vi "HEWH Populate Test Pattern Cluster.vi"(8 "Error In":errorcluster, 11 "all rows":string[][](array[string])) -> (0 "Error Out":errorcluster, 3 "Cluster":T1={"Sequence #"=0.0, "Cycles"=0, "Mode Setting"="", "Flow Rate (GPM)"=0.0, "Temperature (F)"=0.0, "Reset Timer"=FALSE, "Use Temp Decline Method"=FALSE, "Terminate Condition"=enum."C1-Terminate Draw @ Gallon Mark", "Condition Value #1"=0.0, "UE"=FALSE, "LE"=FALSE, "Comp"=FALSE, "Fan"=FALSE, "Test End Time (Sec)"=0.0, "Purge Until Cutout"=FALSE, "Start Conditions"=enum."Heat Source Cutout", "Condition Value #2"=0.0, "Remove Power"=FALSE, "Time"=0.0, "Check Special Cond."=enum."SC1-Do Nothing", "Condition#"=enum."C1", "Draw Flags"=enum."N/A", "Data Processing Delay (FHD 15sec, UEF 5 Sec)"=0.0, "Test Complete"=FALSE} {"Time" format="%<%H:%M:%S>t"})   [LabVIEW 2016]
uses:
  Type Definitions/PRAT Test.ctl
  Utility/Save File/File Setup (Public)/Type Definition/Save File HEWH Heating Control Mode.ctl
  Draw Water Specific/Type Definitions/Terminate Draw Conditions.ctl
  Type Definitions/HEWH Start Conditions.ctl
  Draw Water Specific/Type Definitions/Check Special Condtions.ctl
  Draw Water Specific/Type Definitions/HEWH Special Condition Check.ctl
  Type Definitions/HEWH Draw Flag ENUM.ctl
  Utility/Save File/File Setup.lvlib
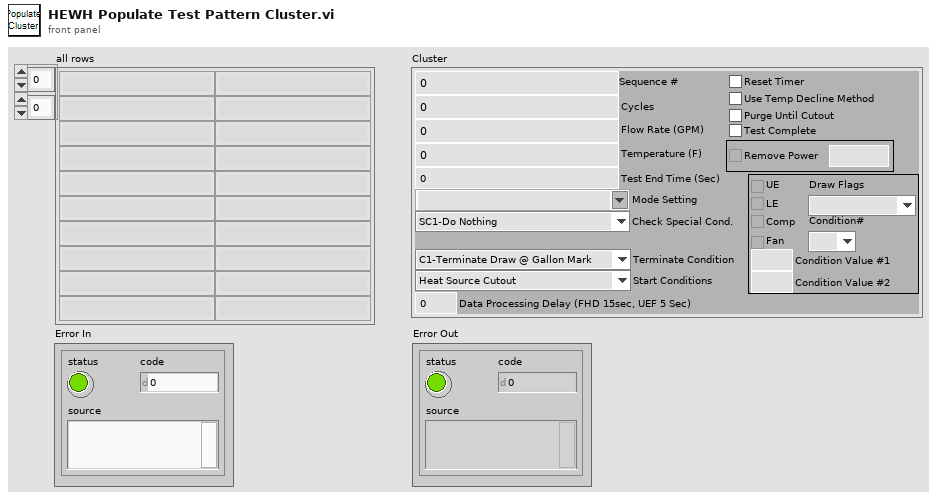
[diagram p1: front panel]
types:
  T1 = typedef "PRAT Test.ctl" = cluster{"Sequence #":dbl, "Cycles":i32, "Mode Setting":T2, "Flow Rate (GPM)":dbl, "Temperature (F)":dbl, "Reset Timer":bool, "Use Temp Decline Method":bool, "Terminate Condition":T3, "Condition Value #1":dbl, "UE":bool, "LE":bool, "Comp":bool, "Fan":bool, "Test End Time (Sec)":dbl, "Purge Until Cutout":bool, "Start Conditions":T4, "Condition Value #2":dbl, "Remove Power":bool, "Time":dbl, "Check Special Cond.":T5, "Condition#":T6, "Draw Flags":T7, "Data Processing Delay (FHD 15sec, UEF 5 Sec)":dbl, "Test Complete":bool}
  T2 = typedef "File Setup.lvlib/Save File HEWH Heating Control Mode.ctl" = string
  T3 = typedef "Terminate Draw Conditions.ctl" = enum16{"C1-Terminate Draw @ Gallon Mark", "C2-Special Last Draw (HU Test)", "C3-RTD Out <=", "C4-Mean Tank Temp <=", "C5-Decrease RTD Out (Deg F)", "C6-Time (Seconds)", "C7-Until Any Heat Source", "C8-Specific Heat Source", "C9-Do Nothing"}
  T4 = typedef "HEWH Start Conditions.ctl" = enum16{"Heat Source Cutout", "At Time (Seconds)", "Every X (Seconds)", "T2 >= X° Below Setpoint", "Seconds From Complete", "Wait for LE & Comp Cutout", "Wait for Comp Cutout", "Wait for LE Cutout", "Wait for UE Cutout"}
  T5 = typedef "Check Special Condtions.ctl" = enum16{"SC1-Do Nothing", "SC2-Check Heat Source (On-C2/Off-C1)", "SC3-Check Skip Condition", "SC4-Check Heat Source ON/Fail"}
  T6 = typedef "HEWH Special Condition Check.ctl" = enum16{"N/A", "C1", "C2", "Reset/Fail", "Skip Draw Sequence"}
  T7 = typedef "HEWH Draw Flag ENUM.ctl" = enum16{"N/A", "None(0)", "Sml(1)", "Med(2)", "SmlMed(3)", "Lrg(4)", "SmlLrg(5)", "MedLrg(6)", "SmlMedLrg(7)"}
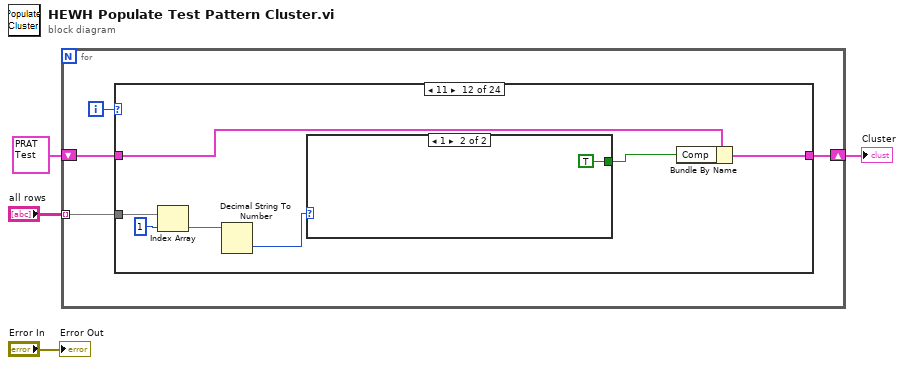
[diagram p0: block diagram]
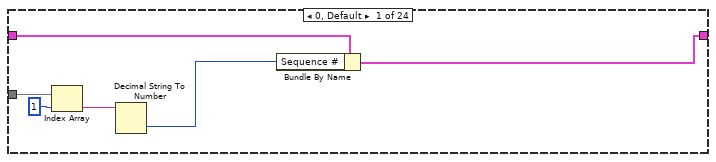
[diagram p2: hidden frame]
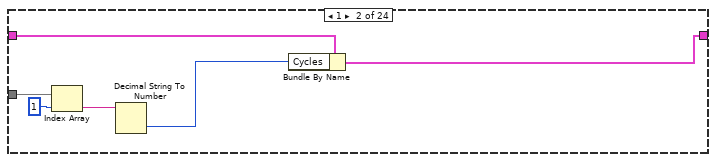
[diagram p3: hidden frame]
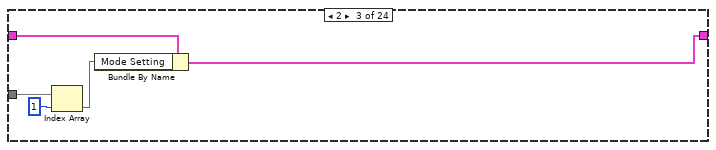
[diagram p4: hidden frame]
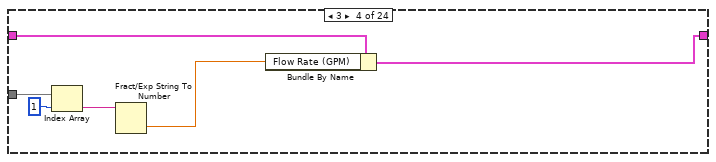
[diagram p5: hidden frame]
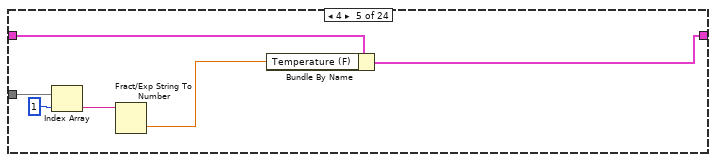
[diagram p6: hidden frame]
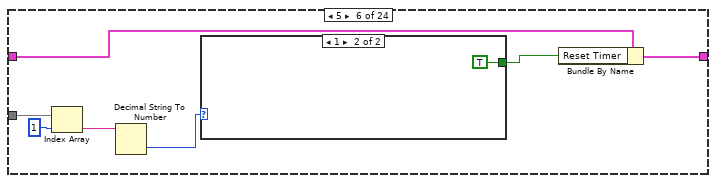
[diagram p7: hidden frame]
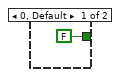
[diagram p8: hidden frame]
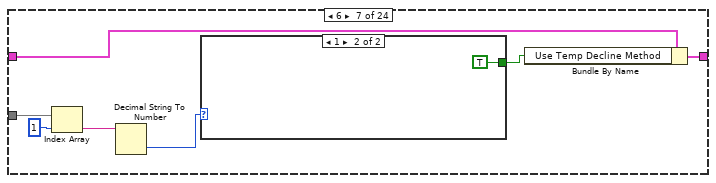
[diagram p9: hidden frame]
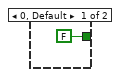
[diagram p10: hidden frame]
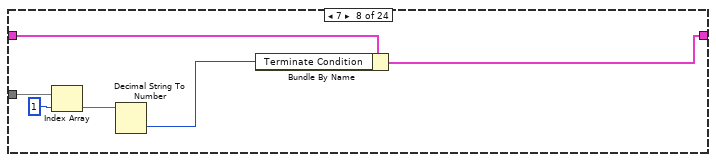
[diagram p11: hidden frame]
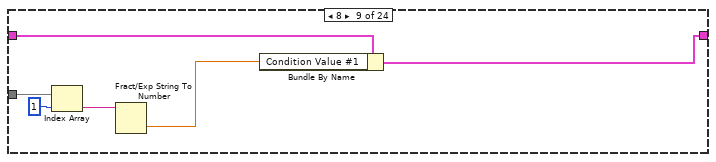
[diagram p12: hidden frame]
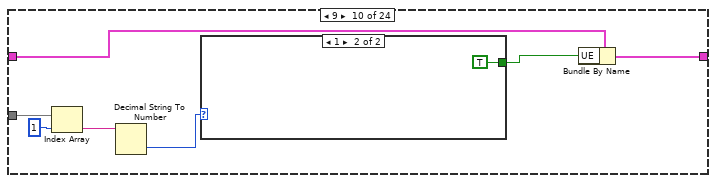
[diagram p13: hidden frame]
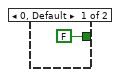
[diagram p14: hidden frame]
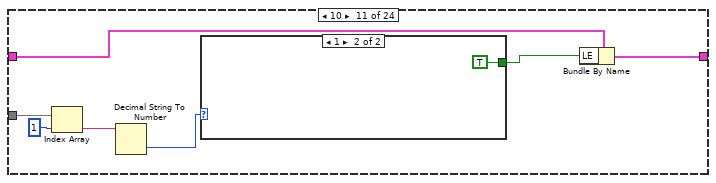
[diagram p15: hidden frame]
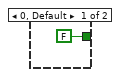
[diagram p16: hidden frame]
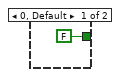
[diagram p17: hidden frame]
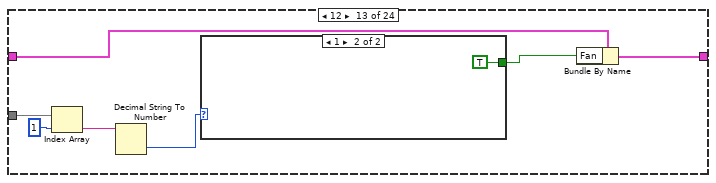
[diagram p18: hidden frame]
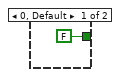
[diagram p19: hidden frame]
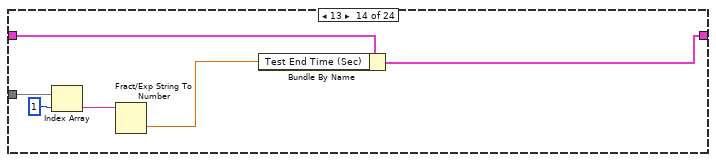
[diagram p20: hidden frame]
diagram:
  n1 = for {
    tunnel: "all rows" -> [w5] mode=indexing
    shift-right: [w6] -> w3
    shift-left: T1 {"Sequence #"=1.0, "Cycles"=1, "Mode Setting"="", "Flow Rate (GPM)"=3.0, "Temperature (F)"=58.0, "Reset Timer"=FALSE, "Use Temp Decline Method"=FALSE, "Terminate Condition"=enum."C9-Do Nothing", "Condition Value #1"=0.0, "UE"=FALSE, "LE"=FALSE, "Comp"=FALSE, "Fan"=FALSE, "Test End Time (Sec)"=0.0, "Purge Until Cutout"=FALSE, "Start Conditions"=enum."Heat Source Cutout", "Condition Value #2"=0.0, "Remove Power"=FALSE, "Time"=82800.0, "Check Special Cond."=enum."SC1-Do Nothing", "Condition#"=enum."N/A", "Draw Flags"=enum."N/A", "Data Processing Delay (FHD 15sec, UEF 5 Sec)"=5.0, "Test Complete"=FALSE} ("Cluster") -> [w7]
    i -> [w8]
    n2 = case shown="11" w8 {
      tunnel: w7 -> [w14 w17 w24 w29 w34 w43 w49 w59 w66 w73 w79 w88 w97 w108 w114 w122 w128 w133 w144 w150 w153 w159 w168 w174]
      tunnel: [w13 w16 w22 w28 w33 w42 w47 w57 w64 w71 w78 w87 w95 w107 w113 w121 w127 w131 w142 w148 w152 w158 w167 w173] -> w6
      tunnel: w5 -> [w12 w15 w23 w30 w32 w41 w48 w58 w65 w72 w80 w86 w96 w106 w115 w120 w129 w132 w143 w149 w154 w160 w166 w175]
      frame 0, Default {
        n3 = Index Array(array=w12, index=1) -> (element=w10:string)
        n4 = Decimal String To Number(string=w10) -> (number=w9:i32)  [unwired: 2 in, 1 out]
        n5 = Bundle By Name(cluster=w14, "Sequence #"=w9) -> (w13:T1)
      }
      frame 1 {
        n6 = Index Array(array=w15, index=1) -> (element=w19:string)
        n7 = Decimal String To Number(string=w19) -> (number=w18:i32)  [unwired: 2 in, 1 out]
        n8 = Bundle By Name(cluster=w17, "Cycles"=w18) -> (w16:T1)
      }
      frame 2 {
        n9 = Index Array(array=w23, index=1) -> (element=w21:string)
        n10 = Bundle By Name(cluster=w24, "Mode Setting"=w21) -> (w22:T1)
      }
      frame 3 {
        n11 = Index Array(array=w30, index=1) -> (element=w27:string)
        n12 = Fract/Exp String To Number(string=w27) -> (number=w26:dbl)  [unwired: 3 in, 1 out]
        n13 = Bundle By Name(cluster=w29, "Flow Rate (GPM)"=w26) -> (w28:T1)
      }
      frame 4 {
        n14 = Index Array(array=w32, index=1) -> (element=w36:string)
        n15 = Fract/Exp String To Number(string=w36) -> (number=w35:dbl)  [unwired: 3 in, 1 out]
        n16 = Bundle By Name(cluster=w34, "Temperature (F)"=w35) -> (w33:T1)
      }
      frame 5 {
        n17 = Index Array(array=w41, index=1) -> (element=w40:string)
        n18 = Decimal String To Number(string=w40) -> (number=w39:i32)  [unwired: 2 in, 1 out]
        n19 = case shown="1" w39 {
          tunnel: [FALSE TRUE] -> w38
          frame 0, Default {
          }
          frame 1 {
          }
        }
        n20 = Bundle By Name(cluster=w43, "Reset Timer"=w38) -> (w42:T1)
      }
      frame 6 {
        n21 = Index Array(array=w48, index=1) -> (element=w52:string)
        n22 = Decimal String To Number(string=w52) -> (number=w51:i32)  [unwired: 2 in, 1 out]
        n23 = case shown="1" w51 {
          tunnel: [FALSE TRUE] -> w50
          frame 0, Default {
          }
          frame 1 {
          }
        }
        n24 = Bundle By Name(cluster=w49, "Use Temp Decline Method"=w50) -> (w47:T1)
      }
      frame 7 {
        n25 = Index Array(array=w58, index=1) -> (element=w60:string)
        n26 = Decimal String To Number(string=w60) -> (number=w56:i32)  [unwired: 2 in, 1 out]
        n27 = Bundle By Name(cluster=w59, "Terminate Condition"=w56) -> (w57:T1)
      }
      frame 8 {
        n28 = Index Array(array=w65, index=1) -> (element=w63:string)
        n29 = Fract/Exp String To Number(string=w63) -> (number=w62:dbl)  [unwired: 3 in, 1 out]
        n30 = Bundle By Name(cluster=w66, "Condition Value #1"=w62) -> (w64:T1)
      }
      frame 9 {
        n31 = Index Array(array=w72, index=1) -> (element=w69:string)
        n32 = Decimal String To Number(string=w69) -> (number=w70:i32)  [unwired: 2 in, 1 out]
        n33 = case shown="1" w70 {
          tunnel: [FALSE TRUE] -> w68
          frame 0, Default {
          }
          frame 1 {
          }
        }
        n34 = Bundle By Name(cluster=w73, "UE"=w68) -> (w71:T1)
      }
      frame 10 {
        n35 = Index Array(array=w80, index=1) -> (element=w81:string)
        n36 = Decimal String To Number(string=w81) -> (number=w82:i32)  [unwired: 2 in, 1 out]
        n37 = case shown="1" w82 {
          tunnel: [FALSE TRUE] -> w77
          frame 0, Default {
          }
          frame 1 {
          }
        }
        n38 = Bundle By Name(cluster=w79, "LE"=w77) -> (w78:T1)
      }
      frame 11 {
        n39 = Index Array(array=w86, index=1) -> (element=w90:string)
        n40 = Decimal String To Number(string=w90) -> (number=w91:i32)  [unwired: 2 in, 1 out]
        n41 = case shown="1" w91 {
          tunnel: [FALSE TRUE] -> w89
          frame 0, Default {
          }
          frame 1 {
          }
        }
        n42 = Bundle By Name(cluster=w88, "Comp"=w89) -> (w87:T1)
      }
      frame 12 {
        n43 = Index Array(array=w96, index=1) -> (element=w99:string)
        n44 = Decimal String To Number(string=w99) -> (number=w100:i32)  [unwired: 2 in, 1 out]
        n45 = case shown="1" w100 {
          tunnel: [FALSE TRUE] -> w98
          frame 0, Default {
          }
          frame 1 {
          }
        }
        n46 = Bundle By Name(cluster=w97, "Fan"=w98) -> (w95:T1)
      }
      frame 13 {
        n47 = Index Array(array=w106, index=1) -> (element=w105:string)
        n48 = Fract/Exp String To Number(string=w105) -> (number=w104:dbl)  [unwired: 3 in, 1 out]
        n49 = Bundle By Name(cluster=w108, "Test End Time (Sec)"=w104) -> (w107:T1)
      }
      frame 14 {
        n50 = Index Array(array=w115, index=1) -> (element=w111:string)
        n51 = Decimal String To Number(string=w111) -> (number=w112:i32)  [unwired: 2 in, 1 out]
        n52 = case shown="1" w112 {
          tunnel: [FALSE TRUE] -> w110
          frame 0, Default {
          }
          frame 1 {
          }
        }
        n53 = Bundle By Name(cluster=w114, "Purge Until Cutout"=w110) -> (w113:T1)
      }
      frame 15 {
        n54 = Index Array(array=w120, index=1) -> (element=w123:string)
        n55 = Decimal String To Number(string=w123) -> (number=w119:i32)  [unwired: 2 in, 1 out]
        n56 = Bundle By Name(cluster=w122, "Start Conditions"=w119) -> (w121:T1)
      }
      frame 16 {
        n57 = Index Array(array=w129, index=1) -> (element=w126:string)
        n58 = Fract/Exp String To Number(string=w126) -> (number=w125:dbl)  [unwired: 3 in, 1 out]
        n59 = Bundle By Name(cluster=w128, "Condition Value #2"=w125) -> (w127:T1)
      }
      frame 17 {
        n60 = Index Array(array=w132, index=1) -> (element=w135:string)
        n61 = Decimal String To Number(string=w135) -> (number=w136:i32)  [unwired: 2 in, 1 out]
        n62 = case shown="1" w136 {
          tunnel: [FALSE TRUE] -> w134
          frame 0, Default {
          }
          frame 1 {
          }
        }
        n63 = Bundle By Name(cluster=w133, "Remove Power"=w134) -> (w131:T1)
      }
      frame 18 {
        n64 = Index Array(array=w143, index=1) -> (element=w141:string)
        n65 = Fract/Exp String To Number(string=w141) -> (number=w140:dbl)  [unwired: 3 in, 1 out]
        n66 = Bundle By Name(cluster=w144, "Time"=w140) -> (w142:T1)
      }
      frame 19 {
        n67 = Index Array(array=w149, index=1) -> (element=w147:string)
        n68 = Decimal String To Number(string=w147) -> (number=w146:i32)  [unwired: 2 in, 1 out]
        n69 = Bundle By Name(cluster=w150, "Check Special Cond."=w146) -> (w148:T1)
      }
      frame 20 {
        n70 = Index Array(array=w154, index=1) -> (element=w156:string)
        n71 = Decimal String To Number(string=w156) -> (number=w155:i32)  [unwired: 2 in, 1 out]
        n72 = Bundle By Name(cluster=w153, "Condition#"=w155) -> (w152:T1)
      }
      frame 21 {
        n73 = Index Array(array=w160, index=1) -> (element=w162:string)
        n74 = Decimal String To Number(string=w162) -> (number=w161:i32)  [unwired: 2 in, 1 out]
        n75 = Bundle By Name(cluster=w159, "Draw Flags"=w161) -> (w158:T1)
      }
      frame 22 {
        n76 = Index Array(array=w166, index=1) -> (element=w165:string)
        n77 = Fract/Exp String To Number(string=w165) -> (number=w164:dbl)  [unwired: 3 in, 1 out]
        n78 = Bundle By Name(cluster=w168, "Data Processing Delay (FHD 15sec, UEF 5 Sec)"=w164) -> (w167:T1)
      }
      frame 23 {
        n79 = Index Array(array=w175, index=1) -> (element=w171:string)
        n80 = Decimal String To Number(string=w171) -> (number=w172:i32)  [unwired: 2 in, 1 out]
        n81 = case shown="1" w172 {
          tunnel: [FALSE TRUE] -> w170
          frame 0, Default {
          }
          frame 1 {
          }
        }
        n82 = Bundle By Name(cluster=w174, "Test Complete"=w170) -> (w173:T1)
      }
    }
  }
  "Cluster" <- w3
  "Error Out" <- "Error In"
